vi "Formul node örneği.vi"() -> ()   [LabVIEW 2014]
panel:
  out "X":dbl
  in  "C":dbl
  in  "B":dbl
  in  "A":dbl
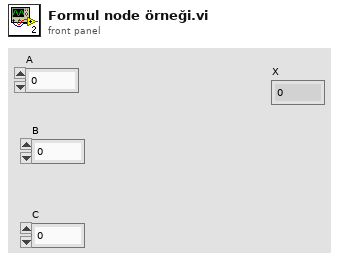
[diagram p1: front panel]
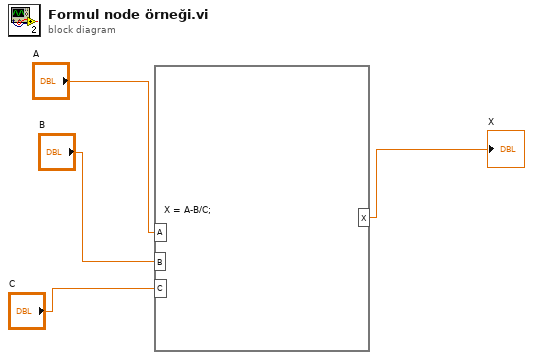
[diagram p0: block diagram]
diagram:
  n1 = formula code="X = A-B/C;"("C"="C", "B"="B", "A"="A") -> ("X"=→"X":dbl)
